vi "Decompose Array - 2D Array - Returns All Elements.vi"() -> ()   [LabVIEW 2017, in "Composition.Tests.lvlib"]
uses:
  Composition.Tests.lvlib
  <vilib>/addons/_JKI Toolkits/Caraya/classes/Assert/Assert Equal Value_Variant.vi
  <vilib>/addons/_JKI Toolkits/Caraya/classes/Assert/Assert Not Error.vi
  <vilib>/addons/_JKI Toolkits/Caraya/classes/Test/Test.lvclass
  Composition/Composition.lvlib
  <vilib>/addons/_JKI Toolkits/Caraya/classes/Assert/Assert.lvclass
panel:
  out "error out":errorcluster
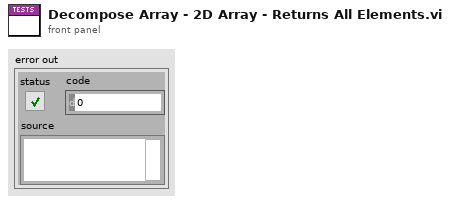
[diagram p1: front panel]
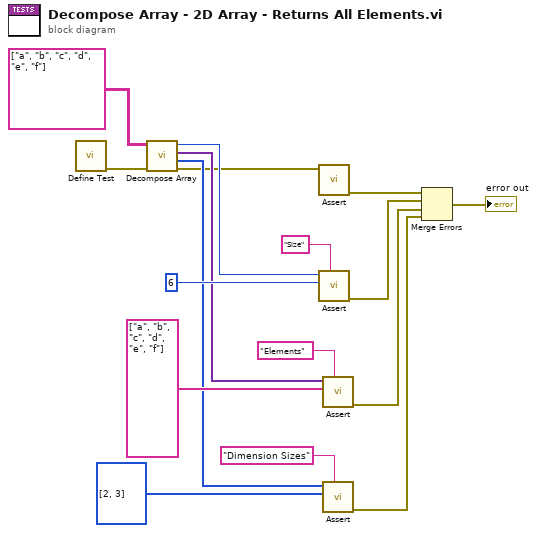
[diagram p0: block diagram]
diagram:
  n1 = call <vilib>:"Define Test.vi"() -> ("error out"=w16:errorcluster)  [unwired: 10 in, 1 out]
  n2 = call "Decompose Array.vi"("error in (no error)"=w16, "Variant Array"=string[][] [["a", "b", "c"], ["d", "e", "f"]]) -> ("error out"=w2:errorcluster, "Dimension Sizes"=w3:i32[], "Elements"=w13:variant[], "Size"=w15:i32)  [unwired: 6 in]
  n3 = call-poly <vilib>:"Assert.vi"("Not Error?"=w2) -> ("error out"=w1:errorcluster)  [unwired: 9 in, 1 out]
  n4 = call-poly <vilib>:"Assert.vi"("Label"="Size", "Y"=6 ("Size"), "X"=w15) -> ("error out"=w11:errorcluster)  [unwired: 7 in, 1 out]
  n5 = call-poly <vilib>:"Assert.vi"("Label"="Elements", "Y"=string[] ["a", "b", "c", "d", "e", "f"], "X"=w13) -> ("error out"=w10:errorcluster)  [unwired: 7 in, 1 out]
  n6 = call-poly <vilib>:"Assert.vi"("Label"="Dimension Sizes", "Y"=i32[] [2, 3] ("Dimension Sizes"), "X"=w3) -> ("error out"=w4:errorcluster)  [unwired: 7 in, 1 out]
  n7 = Merge Errors(w1, w11, w10, w4) -> (→"error out":errorcluster)
